vi "sub_5li_TabloBoya.vi"(2 "Table in":refnum<vi>, 3 "Tablo Degerleri":dbl[][](array[numeric])) -> (0 "Test Result":bool, 1 "RESULTS":string[](array[string]))   [LabVIEW 2014]
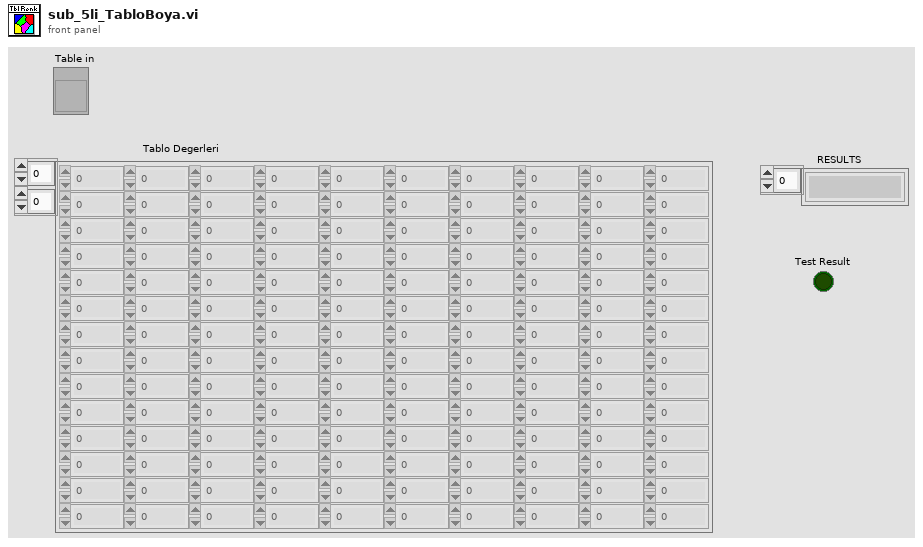
[diagram p1: front panel]
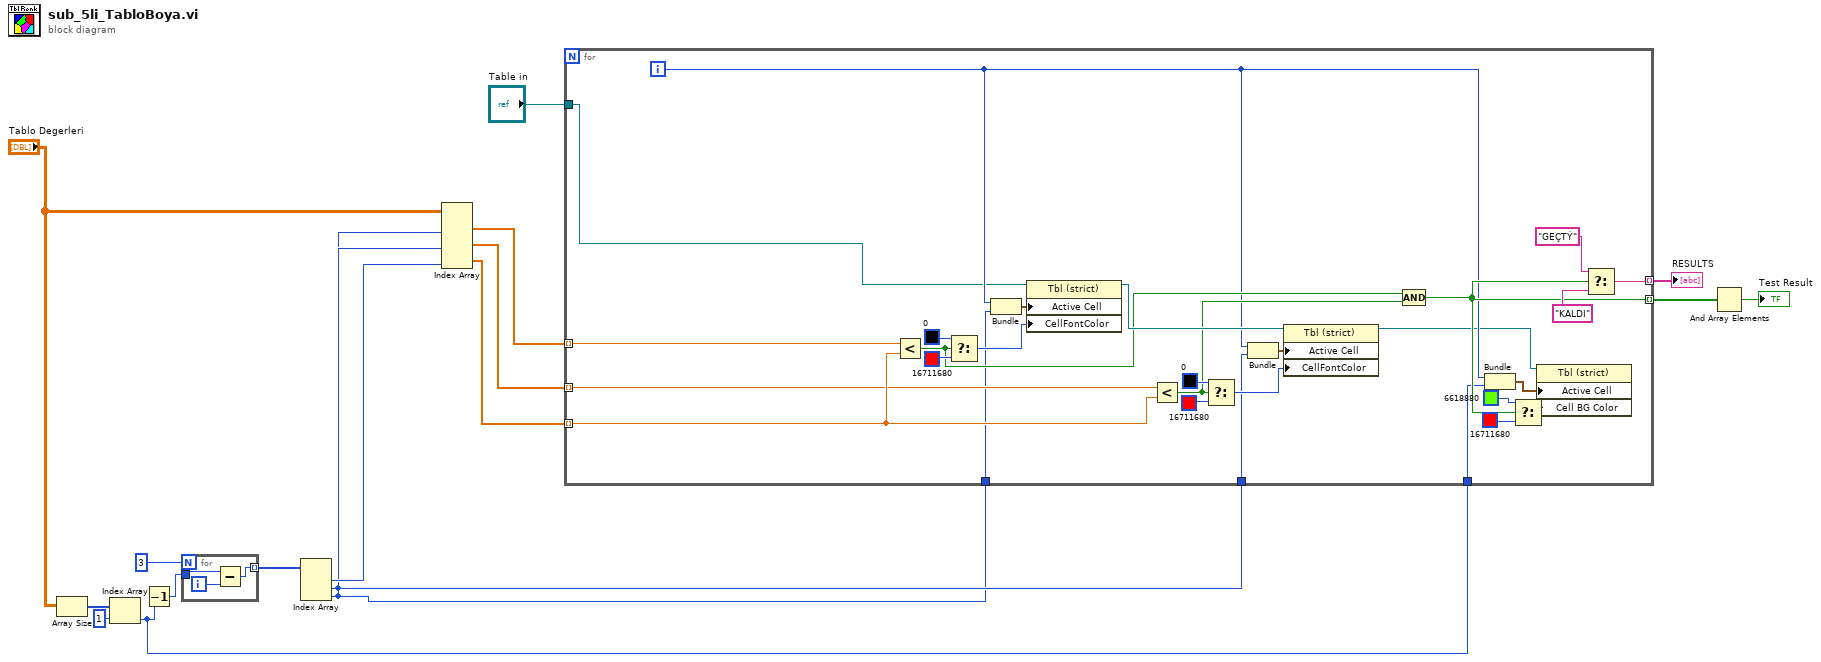
[diagram p0: block diagram]
diagram:
  n1 = Array Size(array="Tablo Degerleri") -> (size(s)=w9:i32[])
  n2 = Index Array(array=w9, index=1) -> (element=w3:i32)
  n3 = Decrement(x=w3) -> (x-1=w4:i32)
  n4 = for {
    N: 3 -> [_]
    tunnel: [w18] -> w7 mode=indexing
    tunnel: w4 -> [w19]
    i -> [w20]
    n5 = Subtract(x=w19, y=w20) -> (x-y=w18:i32)
  }
  n6 = Index Array(array=w7) -> (element #1=w5:i32, element #2=w2:i32, element #3=w1:i32)  [unwired: 3 in]
  n7 = Index Array(array="Tablo Degerleri", index (col) #1=w1, index (col) #2=w2, index (col) #3=w5) -> (element #1=w16:dbl[], element #2=w15:dbl[], element #3=w14:dbl[])  [unwired: 3 in]
  n8 = for {
    tunnel: "Table in" -> [w21]
    tunnel: w16 -> [w44] mode=indexing
    tunnel: w15 -> [w37] mode=indexing
    tunnel: w14 -> [w38] mode=indexing
    tunnel: [w32] -> w13 mode=indexing
    tunnel: [w31] -> w12 mode=indexing
    tunnel: w3 -> [w24]
    tunnel: w2 -> [w23]
    tunnel: w1 -> [w22]
    i -> [w27]
    n9 = Less?(x=w44, y=w38) -> (x < y?=w35:bool)
    n10 = Select(t=u32 0, s=w35, f=u32 16711680) -> (s? t:f=w46:u32)
    n11 = Bundle(w27, w22) -> (w45:cluster{i32, i32})  [unwired: 1 in]
    n12 = property on="Property Node" class="Tbl (strict)"(reference=w21, "Active Cell"=w45, "CellFontColor"=w46) -> (reference out=w39:refnum<vi>)  [unwired: 1 in, 1 out]
    n13 = Less?(x=w37, y=w38) -> (x < y?=w36:bool)
    n14 = Select(t=u32 0, s=w36, f=u32 16711680) -> (s? t:f=w41:u32)
    n15 = Bundle(w27, w23) -> (w40:cluster{i32, i32})  [unwired: 1 in]
    n16 = property on="Property Node" class="Tbl (strict)"(reference=w39, "Active Cell"=w40, "CellFontColor"=w41) -> (reference out=w25:refnum<vi>)  [unwired: 1 in, 1 out]
    n17 = Compound Arithmetic op=AND(w35, w36) -> (w31:bool)
    n18 = Bundle(w27, w24) -> (w26:cluster{i32, i32})  [unwired: 1 in]
    n19 = Select(t=u32 6618880, s=w31, f=u32 16711680) -> (s? t:f=w28:u32)
    n20 = property on="Property Node" class="Tbl (strict)"(reference=w25, "Active Cell"=w26, "Cell BG Color"=w28) -> ()  [unwired: 1 in, 2 out]
    n21 = Select(t="GEÇTÝ", s=w31, f="KALDI") -> (s? t:f=w32:string)
  }
  "RESULTS" <- w13
  n22 = And Array Elements(Boolean array=w12) -> (logical AND=→"Test Result":bool)
